vi "windows_keyboard_event.vi"(8 "error in (no error)":errorcluster, 11 "String to write via keyboard emulation, never empty":string) -> (0 "error out":errorcluster, 3 "vi path (only on error)":path)   [LabVIEW 2011]
uses:
  user32.dll
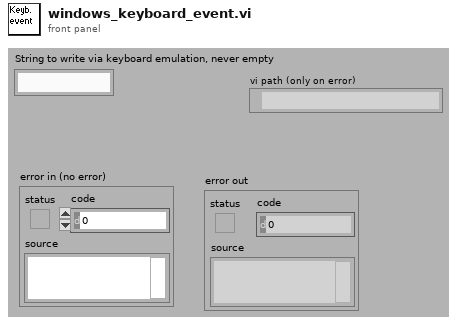
[diagram p1: front panel]
types:
  T1 = cluster{"return type":u32, "KEYEVENTF_KEYUP":i32}
  T2 = cluster{"return type":u32, "KEYEVENTF_KEYUP":i32}[]
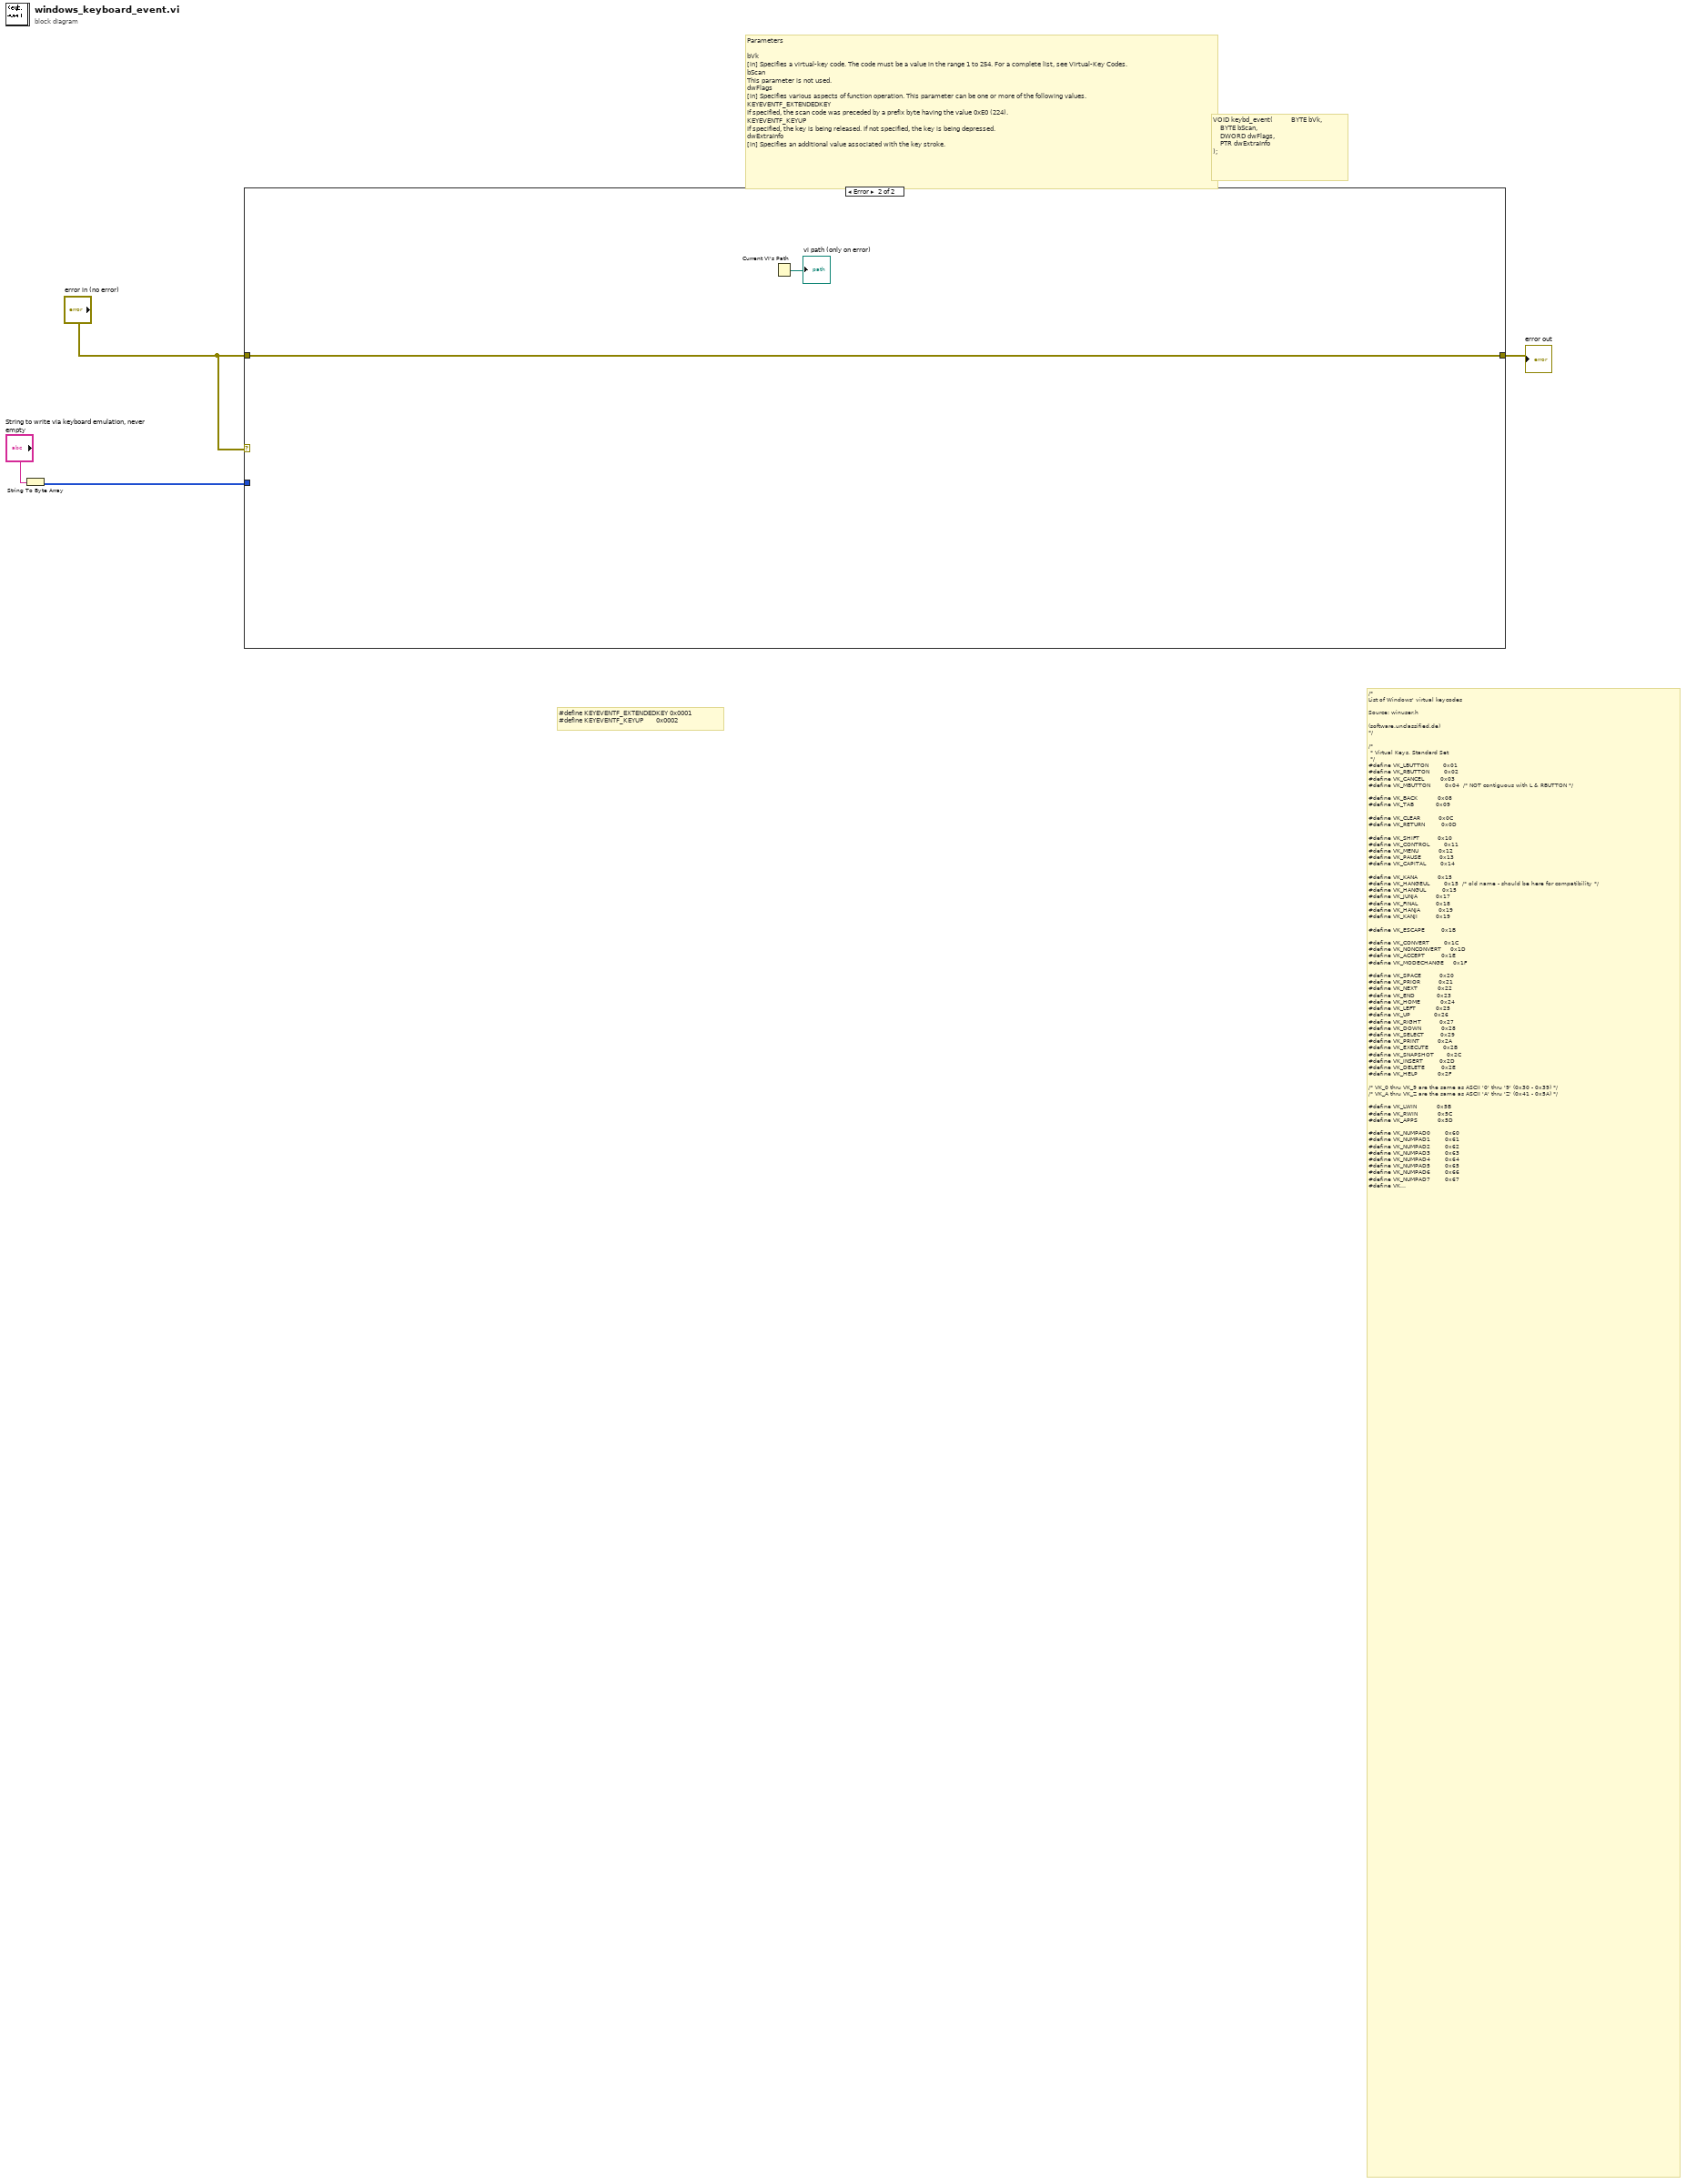
[diagram p0: block diagram]
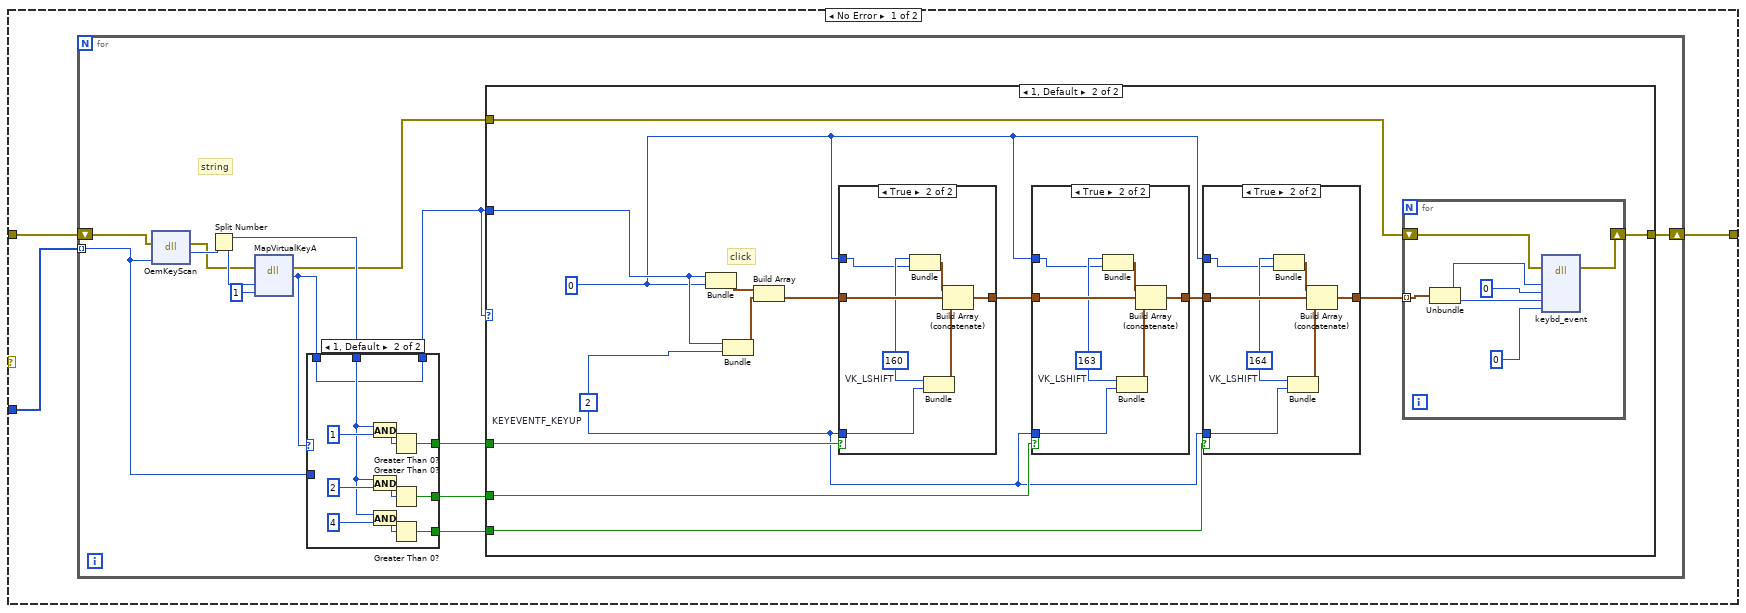
[diagram p2: hidden frame]
diagram:
  # "#define KEYEVENTF_EXTENDEDKEY 0x0001\n#define KEYEVENTF_KEYUP       0x0002"
  # "/*\nList of Windows' virtual keycodes\n \nSource: winuser.h\n \n(software.unclassified.de)\n*/\n \n/*\n * Virtual Keys, Standard Set\n */\n#define VK_LBUTTON        0x01\n#define VK_RBUTTON        0x02\n#define VK_CANCEL         0x03\n#define VK_MBUTTON        0x04  /* NOT contiguous with L & RBUTTON */\n \n#define VK_BACK           0x08\n#define VK_TAB            0x09\n \n#define VK_CLEAR          0x0C\n#define VK_RETURN         0x0D\n \n#define VK_SHIFT          0x10\n#define VK_CONTROL        0x11\n#define VK_MENU           0x12\n#define VK_PAUSE          0x13\n#define VK_CAPITAL        0x14\n \n#define VK_KANA           0x15\n#define VK_HANGEUL        0x15  /* old name - should be here for compatibility */\n#define VK_HANGUL         0x15\n#define VK_JUNJA          0x17\n#define VK_FINAL          0x18\n#define VK_HANJA          0x19\n#define VK_KANJI          0x19\n \n#define VK_ESCAPE         0x1B\n \n#define VK_CONVERT        0x1C\n#define VK_NONCONVERT     0x1D\n#define VK_ACCEPT         0x1E\n#define VK_MODECHANGE     0x1F\n \n#define VK_SPACE          0x20\n#define VK_PRIOR          0x21\n#define VK_NEXT           0x22\n#define VK_END            0x23\n#define VK_HOME           0x24\n#define VK_LEFT           0x25\n#define VK_UP             0x26\n#define VK_RIGHT          0x27\n#define VK_DOWN           0x28\n#define VK_SELECT         0x29\n#define VK_PRINT          0x2A\n#define VK_EXECUTE        0x2B\n#define VK_SNAPSHOT       0x2C\n#define VK_INSERT         0x2D\n#define VK_DELETE         0x2E\n#define VK_HELP           0x2F\n \n/* VK_0 thru VK_9 are the same as ASCII '0' thru '9' (0x30 - 0x39) */\n/* VK_A thru VK_Z are the same as ASCII 'A' thru 'Z' (0x41 - 0x5A) */\n \n#define VK_LWIN           0x5B\n#define VK_RWIN           0x5C\n#define VK_APPS           0x5D\n \n#define VK_NUMPAD0        0x60\n#define VK_NUMPAD1        0x61\n#define VK_NUMPAD2        0x62\n#define VK_NUMPAD3        0x63\n#define VK_NUMPAD4        0x64\n#define VK_NUMPAD5        0x65\n#define VK_NUMPAD6        0x66\n#define VK_NUMPAD7        0x67\n#define VK_NUMPAD8        0x68\n#define VK_NUMPAD9        0x69\n#define VK_MULTIPLY       0x6A\n#define VK_ADD            0x6B\n#define VK_SEPARATOR      0x6C\n#define VK_SUBTRACT       0x6D\n#define VK_DECIMAL        0x6E\n#define VK_DIVIDE         0x6F\n#define VK_F1             0x70\n#define VK_F2             0x71\n#define VK_F3             0x72\n#define VK_F4             0x73\n#define VK_F5             0x74\n#define VK_F6             0x75\n#define VK_F7             0x76\n#define VK_F8             0x77\n#define VK_F9             0x78\n#define VK_F10            0x79\n#define VK_F11            0x7A\n#define VK_F12            0x7B\n#define VK_F13            0x7C\n#define VK_F14            0x7D\n#define VK_F15            0x7E\n#define VK_F16            0x7F\n#define VK_F17            0x80\n#define VK_F18            0x81\n#define VK_F19            0x82\n#define VK_F20            0x83\n#define VK_F21            0x84\n#define VK_F22            0x85\n#define VK_F23            0x86\n#define VK_F24            0x87\n \n#define VK_NUMLOCK        0x90\n#define VK_SCROLL         0x91\n \n/*\n * VK_L* & VK_R* - left and right Alt, Ctrl and Shift virtual keys.\n * Used only as parameters to GetAsyncKeyState() and GetKeyState().\n * No other API or message will distinguish left and right keys in this way.\n */\n#define VK_LSHIFT         0xA0\n#define VK_RSHIFT         0xA1\n#define VK_LCONTROL       0xA2\n#define VK_RCONTROL       0xA3\n#define VK_LMENU          0xA4\n#define VK_RMENU          0xA5\n \n#if(WINVER >= 0x0400)\n#define VK_PROCESSKEY     0xE5\n#endif /* WINVER >= 0x0400 */\n \n#define VK_ATTN           0xF6\n#define VK_CRSEL          0xF7\n#define VK_EXSEL          0xF8\n#define VK_EREOF          0xF9\n#define VK_PLAY           0xFA\n#define VK_ZOOM           0xFB\n#define VK_NONAME         0xFC\n#define VK_PA1            0xFD\n#define VK_OEM_CLEAR      0xFE"
  # "Parameters\n\nbVk\n[in] Specifies a virtual-key code. The code must be a value in the range 1 to 254. For a complete list, see Virtual-Key Codes. \nbScan\nThis parameter is not used. \ndwFlags\n[in] Specifies various aspects of function operation. This parameter can be one or more of the following values. \nKEYEVENTF_EXTENDEDKEY\nIf specified, the scan code was preceded by a prefix byte having the value 0xE0 (224).\nKEYEVENTF_KEYUP\nIf specified, the key is being released. If not specified, the key is being depressed.\ndwExtraInfo\n[in] Specifies an additional value associated with the key stroke."
  # "VOID keybd_event(          BYTE bVk,\n    BYTE bScan,\n    DWORD dwFlags,\n    PTR dwExtraInfo\n);"
  n1 = String To Byte Array(string="String to write via keyboard emulation, never empty") -> (unsigned byte array=w3:u8[])
  n2 = case shown="Error" "error in (no error)" {
    tunnel: w3 -> [w7 _]
    tunnel: "error in (no error)" -> [w6 w81]
    tunnel: [w5 w81] -> w2
    frame No Error {
      n3 = for {
        tunnel: w7 -> [w21] mode=indexing
        shift-right: [w8] -> w5
        shift-left: w6 -> [w11]
        # "string"
        n4 = dll-call lib="user32.dll" fn="OemKeyScan"(error in=w11, "wOemChar"=w21) -> (error out=w10:errorcluster, "return type"=w15:u32)  [unwired: 2 in, 2 out]
        n5 = Split Number(x=w15) -> (hi(x)=w13:u16, lo(x)=w14:u16)
        n6 = dll-call lib="user32.dll" fn="MapVirtualKeyA"(error in=w10, "uCode"=w14, "uMapType"=u32 1) -> (error out=w9:errorcluster, "return type"=w12:u32)  [unwired: 3 in, 2 out]
        n7 = case shown="1, Default" w12 {
          tunnel: [_ w31] -> w20
          tunnel: [_ w28] -> w19
          tunnel: w13 -> [_ w25]
          tunnel: [_ w24] -> w18
          tunnel: [w22 w23] -> w17
          tunnel: w21 -> [w22 _]
          tunnel: w12 -> [_ w23]
          frame 0 {
          }
          frame 1, Default {
            n8 = And(x=w25, y=u16 1) -> (x .and. y?=w33:u16)
            n9 = And(x=w25, y=u16 2) -> (x .and. y?=w29:u16)
            n10 = And(x=w25, y=u16 4) -> (x .and. y?=w27:u16)
            n11 = Greater Than 0?(x=w33) -> (x > 0?=w31:bool)
            n12 = Greater Than 0?(x=w29) -> (x > 0?=w28:bool)
            n13 = Greater Than 0?(x=w27) -> (x > 0?=w24:bool)
          }
        }
        n14 = case shown="1, Default" w17 {
          tunnel: w20 -> [_ w48]
          tunnel: w17 -> [_ w46]
          tunnel: w19 -> [_ w44]
          tunnel: w18 -> [_ w39]
          tunnel: w9 -> [w34 w36]
          tunnel: [w34 w35] -> w8
          frame 0 {
          }
          frame 1, Default {
            w41 = 0 ("dwFlags")
            w40 = 2  # KEYEVENTF_KEYUP
            # "click"
            n15 = Bundle("return type"=w46, "dwFlags"=w41) -> (w38:cluster{"return type":u32, "dwFlags":i32})  [unwired: 1 out]
            n16 = Bundle("return type"=w46, "KEYEVENTF_KEYUP"=w40) -> (w37:T1)  [unwired: 1 out]
            n17 = Build Array(w38, w37) -> (w47:T2)
            n18 = case shown="True" w48 {
              tunnel: w47 -> [w65 w70]
              tunnel: [w65 w69] -> w45
              tunnel: w41 -> [_ w67]
              tunnel: w40 -> [_ w66]
              frame False {
              }
              frame True {
                w68 = 160  # VK_LSHIFT
                n19 = Bundle("VK_LSHIFT"=w68, "dwFlags"=w67) -> (w71:cluster{"VK_LSHIFT ":i32, "dwFlags":i32})  [unwired: 1 out]
                n20 = Bundle("VK_LSHIFT"=w68, "KEYEVENTF_KEYUP"=w66) -> (w72:cluster{"VK_LSHIFT ":i32, "KEYEVENTF_KEYUP":i32})  [unwired: 1 out]
                n21 = Build Array (concatenate)(w71, w70, w72) -> (w69:T2)
              }
            }
            n22 = case shown="True" w44 {
              tunnel: w45 -> [w57 w62]
              tunnel: [w57 w61] -> w42
              tunnel: w41 -> [_ w59]
              tunnel: w40 -> [_ w58]
              frame False {
              }
              frame True {
                w60 = 163  # VK_LSHIFT
                n23 = Bundle("VK_LSHIFT"=w60, "dwFlags"=w59) -> (w63:cluster{"VK_LSHIFT ":i32, "dwFlags":i32})  [unwired: 1 out]
                n24 = Bundle("VK_LSHIFT"=w60, "KEYEVENTF_KEYUP"=w58) -> (w64:cluster{"VK_LSHIFT ":i32, "KEYEVENTF_KEYUP":i32})  [unwired: 1 out]
                n25 = Build Array (concatenate)(w63, w62, w64) -> (w61:T2)
              }
            }
            n26 = case shown="True" w39 {
              tunnel: w42 -> [w49 w54]
              tunnel: [w49 w53] -> w43
              tunnel: w41 -> [_ w51]
              tunnel: w40 -> [_ w50]
              frame False {
              }
              frame True {
                w52 = 164  # VK_LSHIFT
                n27 = Bundle("VK_LSHIFT"=w52, "dwFlags"=w51) -> (w55:cluster{"VK_LSHIFT ":i32, "dwFlags":i32})  [unwired: 1 out]
                n28 = Bundle("VK_LSHIFT"=w52, "KEYEVENTF_KEYUP"=w50) -> (w56:cluster{"VK_LSHIFT ":i32, "KEYEVENTF_KEYUP":i32})  [unwired: 1 out]
                n29 = Build Array (concatenate)(w55, w54, w56) -> (w53:T2)
              }
            }
            n30 = for {
              tunnel: w43 -> [w77] mode=indexing
              shift-right: [w73] -> w35
              shift-left: w36 -> [w74]
              n31 = Unbundle(w77) -> ("return type"=w76:u32, "KEYEVENTF_KEYUP"=w75:i32)
              n32 = dll-call lib="user32.dll" fn="keybd_event"(error in=w74, "bVk"=w76, "bScan"=u8 0, "dwFlags"=w75, "dwExtraInfo"=0 ("dwFlags")) -> (error out=w73:errorcluster)  [unwired: 5 in, 3 out]
            }
          }
        }
      }
    }
    frame Error {
      n33 = Current VI's Path() -> (path=→"vi path (only on error)":path)
    }
  }
  "error out" <- w2
